vi "Sprite_DecodeRLEToMemory.vi"(11 "Sprite ID":u8) -> ()   [LabVIEW 2020]
uses:
  <vilib>/Utility/error.llb/Clear Errors.vi
  <vilib>/rvi/Emulation/niFpgaSctlEmulationGetInTimedLoop.vi
  <vilib>/rvi/Emulation/niFpgaEmulationIsFPGAContextNoSignature.vi
  <vilib>/rvi/DataTransferAndStorage/Container/Common/niFpgaContainerGetUniqueNameForEmu.vi
  <vilib>/rvi/Memory/Memory_Emulation/niFpgaMemoryEmulationCacheClearOnFirstRun.vi
  <vilib>/rvi/Memory/Memory_Emulation/nirvimemoryEmulationManagerCache_MakeExclusive.vi
  <vilib>/rvi/Memory/Memory_Emulation/niFpgaMemoryEmulationValidateCache.vi
  <vilib>/rvi/Memory/Memory_Emulation/nirvimemoryEmulationManagerCache_InsertValue.vi
  <vilib>/rvi/Memory/Memory_Emulation/nirvimemoryEmulationManagerCache_ReleaseExclusive.vi
  <vilib>/rvi/Memory/Memory_Emulation/nirvimemoryEmulationManagerCache_GetValue.vi
  <vilib>/rvi/Memory/Memory_Emulation/nirvimemoryEmulationManagerCache_SetValue.vi
  <vilib>/rvi/Emulation/niFpgaProcessEmulError.vi
  <vilib>/rvi/Memory/Memory_Emulation/nirvimemoryFastEmulation.vi
  <vilib>/rvi/Memory/Memory_Emulation/nirvimemoryEmulation.vi
  <vilib>/rvi/errors/nirviReportUnexpectedCaseInternalError (U32).vi
  <vilib>/rvi/DataTransferAndStorage/Container/XNode/niFpgaContainer.xnode
  <vilib>/rvi/DataTransferAndStorage/Register/Emulation/niFpgaRegisterEmulation.vi
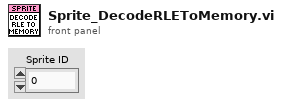
[diagram p1: front panel]
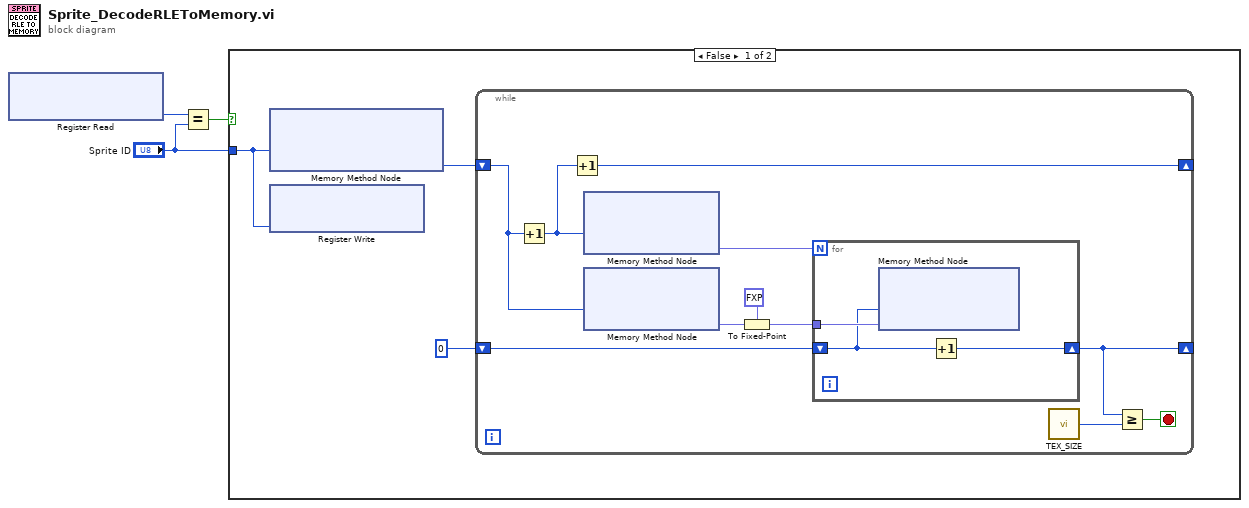
[diagram p0: block diagram]
diagram:
  n1 = xnode "Register Read"() -> ("Data"=w3:u8)  [unwired: 1 in, 1 out]
  n2 = Equal?(x=w3, y="Sprite ID") -> (x = y?=w1:bool)
  n3 = case shown="False" w1 {
    tunnel: "Sprite ID" -> [w4 _]
    frame False {
      n4 = xnode ("Memory Method Node")("Address"=w4) -> ("Data"=w6:u32)  [unwired: 1 in, 1 out]
      n5 = xnode "Register Write"("Data"=w4) -> ()  [unwired: 1 in, 1 out]
      n6 = while {
        shift-right: [w9] -> _
        shift-left: w6 -> [w12]
        shift-right: [w15] -> _
        shift-left: u16 0 -> [w16]
        stop <- w13 stop-if-true
        n7 = Increment(x=w12) -> (x+1=w10:u32)
        n8 = Increment(x=w10) -> (x+1=w9:u32)
        n9 = xnode ("Memory Method Node")("Address"=w10) -> ("Data"=w11:fxp<+,12,12>)  [unwired: 1 in, 1 out]
        n10 = xnode ("Memory Method Node")("Address"=w12) -> ("Data"=w17:fxp<+,12,12>)  [unwired: 1 in, 1 out]
        n11 = To Fixed-Point(fixed-point type=fxp<+,6,6> 0.0, number=w17) -> (fixed-point=w8:fxp<+,6,6>)
        n12 = for {
          N: w11 -> [_]
          tunnel: w8 -> [w20]
          shift-right: [w18] -> w15
          shift-left: w16 -> [w19]
          n13 = xnode ("Memory Method Node")("Address"=w19, "Data"=w20) -> ()  [unwired: 1 in, 1 out]
          n14 = Increment(x=w19) -> (x+1=w18:u16)
        }
        n15 = call "TEX_SIZE.vi"() -> ("TEX_SIZE"=w14:u32)
        n16 = Greater Or Equal?(x=w15, y=w14) -> (x >= y?=w13:bool)
      }
    }
    frame True {
    }
  }
